vi "CRC判定.vi"(2 "报文":string) -> (10 "功能码":u8, 11 "无符号字节数组":u8[](array[numeric]), 14 "报文输出":string, 18 "CRC正确":bool)   [LabVIEW 2019, in "MainPage.lvlib" / "MainPage.lvclass"]
uses:
  MainPage.lvclass
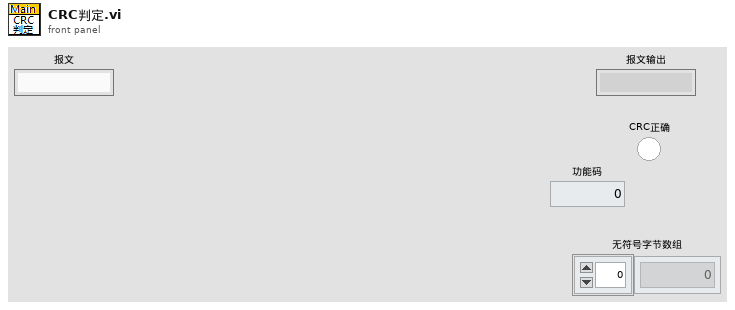
[diagram p1: front panel]
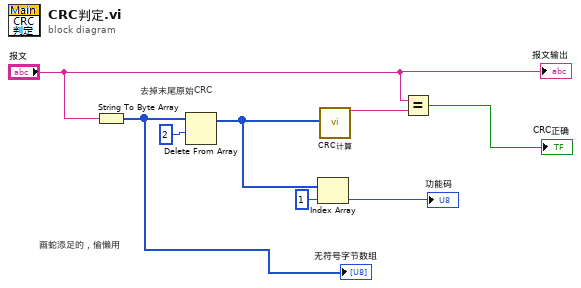
[diagram p0: block diagram]
diagram:
  # "画蛇添足的，偷懒用"
  # "去掉末尾原始CRC"
  n1 = String To Byte Array(string="报文") -> (unsigned byte array=w1:u8[])
  "无符号字节数组" <- w1
  n2 = Delete From Array(array=w1, length=2 ("长度")) -> (array with subset deleted=w4:u8[])  [unwired: 1 in, 1 out]
  n3 = Index Array(array=w4, index=1 ("索引")) -> (element=→"功能码":u8)
  n4 = call "CRC计算.vi"("无校验U8数组"=w4) -> ("计算后字符串"=w7:string)  [unwired: 17 in, 1 out]
  n5 = Equal?(x="报文", y=w7) -> (x = y?=→"CRC正确":bool)
  "报文输出" <- "报文"
